vi "PrefDialog.vi"(8 "error in (no error)":errorcluster, 11 "MyPluginsBase in":refnum<class "PacificPowerSource.lvclass">) -> (0 "error out":errorcluster, 1 "Save As":bool, 2 "Changed":bool, 3 "MyPluginsBase out":refnum<class "PacificPowerSource.lvclass">)   [LabVIEW 2018, in "AcPwrPlugins.lvlib" / "PacificPowerSource.lvclass"]
doc: "This VI allows the user to load the previous device settings that were stored on disk via a .ini file, overwrite the device settings, and save the current settings to a completely new file."
uses:
  PacificPowerSource.lvclass
  C:/Users/Public/Documents/Projects/NistPluggableModules/AcPwr/AcPwrPlugins/AcPwrBaseClass/AcPwrBase.lvclass
  C:/Program Files (x86)/National Instruments/LabVIEW 2018/user.lib/NIST/BaseClasses/BasePlugin_class/BasePlugin.lvclass
  TypeDefs/LoadSettings.ctl
  TypeDefs/Measurements.ctl
  AcPwrBaseClass/AcPwrBase.lvclass/AcPwrBase.ctl
  FGen/MemberClasses/FunctionBaseClass/FunctionBase.lvclass
  <userlib>/NIST/BaseClasses/BasePlugin_class/BasePlugin.lvclass/BasePlugin.ctl
  AcPwrBaseClass/Accessors/Read RefreshTime.vi
  AcPwrBaseClass/Accessors/Read FunctionClass.vi
  AcPwrBaseClass/Accessors/Write FunctionClass.vi
  AcPwrBaseClass/Accessors/Write FunctionINIFilePath.vi
  <userlib>/NIST/BaseClasses/BasePlugin_class/Accessors/Read PluginIniFilePath.vi
  AcPwrBaseClass/Accessors/Write RefreshTime.vi
  <userlib>/NIST/BaseClasses/BasePlugin_class/Accessors/Write PluginIniFilePath.vi
  <vilib>/Utility/error.llb/Error Cluster From Error Code.vi
  <vilib>/ErrorRing/Error Ring.xnode
  <userlib>/NIST/BaseClasses/Object_class/BaseObject.lvclass
  <vilib>/Utility/config.llb/NI_LVConfig.lvlib
  AcPwrBaseClass/AcPwrBase.lvclass
panel:
  in  "Measurements":T1 {"Measurement Type (0: Voltage RMS L-N)" items=["Voltage RMS L-N", "Voltage RMS L-L", "Frequency", "Current RMS", "Current Peak", "Crest Factor", "Power Factor", "Power VA", "Real Power", "Voltage Harmonic THD", "Voltage Harmonic OHD", "Voltage Harmonic EHD", "Current Harmonic THD", "Current Harmonic OHD", "Current Harmonic EHD"]; "Channel Name(1: A)" items=["A"=1, "B"=2, "C"=3]}
  in  "WaveformIniFilePath":path
  in  "BtnConfigureWaveforms":bool
  in  "btnSaveAs":bool
  in  "RefreshTime":dbl
  in  "btnSave":bool
  in  "btnCancel":bool
  in  "Load Settings":T2 {"Arbitrary Waveform"."Waveform Number (2: Arbitrary Waveform2)" items=["Arbitrary Waveform 2"=2, "Arbitrary Waveform 3"=3, "Arbitrary Waveform 4"=4, "Arbitrary Waveform 5"=5, "Arbitrary Waveform 6"=6, "Arbitrary Waveform 7"=7, "Arbitrary Waveform 8"=8, "Arbitrary Waveform 9"=9, "Arbitrary Waveform 10"=10, "Arbitrary Waveform 11"=11, "Arbitrary Waveform 12"=12, "Arbitrary Waveform 13"=13, "Arbitrary Waveform 14"=14, "Arbitrary Waveform 15"=15, "Arbitrary Waveform 16"=16, "Arbitrary Waveform 17"=17, "Arbitrary Waveform 18"=18, "Arbitrary Waveform 19"=19, "Arbitrary Waveform 20"=20, "Arbitrary Waveform 21"=21, "Arbitrary Waveform 22"=22]; "Waveform"."Waveform (1: Sine)" items=["Sine"=1, "Arbitrary Waveform 2"=2, "Arbitrary Waveform 3"=3, "Arbitrary Waveform 4"=4, "Arbitrary Waveform 5"=5, "Arbitrary Waveform 6"=6, "Arbitrary Waveform 7"=7, "Arbitrary Waveform 8"=8, "Arbitrary Waveform 9"=9, "Arbitrary Waveform 10"=10, "Arbitrary Waveform 11"=11, "Arbitrary Waveform 12"=12, "Arbitrary Waveform 13"=13, "Arbitrary Waveform 14"=14, "Arbitrary Waveform 15"=15, "Arbitrary Waveform 16"=16, "Arbitrary Waveform 17"=17, "Arbitrary Waveform 18"=18, "Arbitrary Waveform 19"=19, "Arbitrary Waveform 20"=20, "Arbitrary Waveform 21"=21, "Arbitrary Waveform 22"=22]; "Waveform"."Channel Name (1: A)" items=["A"=1, "B"=2, "C"=3]; "Frequency"."Frequency Range (600Hz)" items=["150 Hz", "300 Hz", "600 Hz", "1200 Hz"]; "Range Control (0: Auto)" items=["Auto", "<110 V", "110 V -120.9 V", "121 V - 130.9 V", "> 131 V"]; "Configure Output"."Form (3: Three)" items=["Single", "Split", "Three"]; "Configure Output"."Coupling  (0: Direct)" items=["Direct", "Transformer"]}
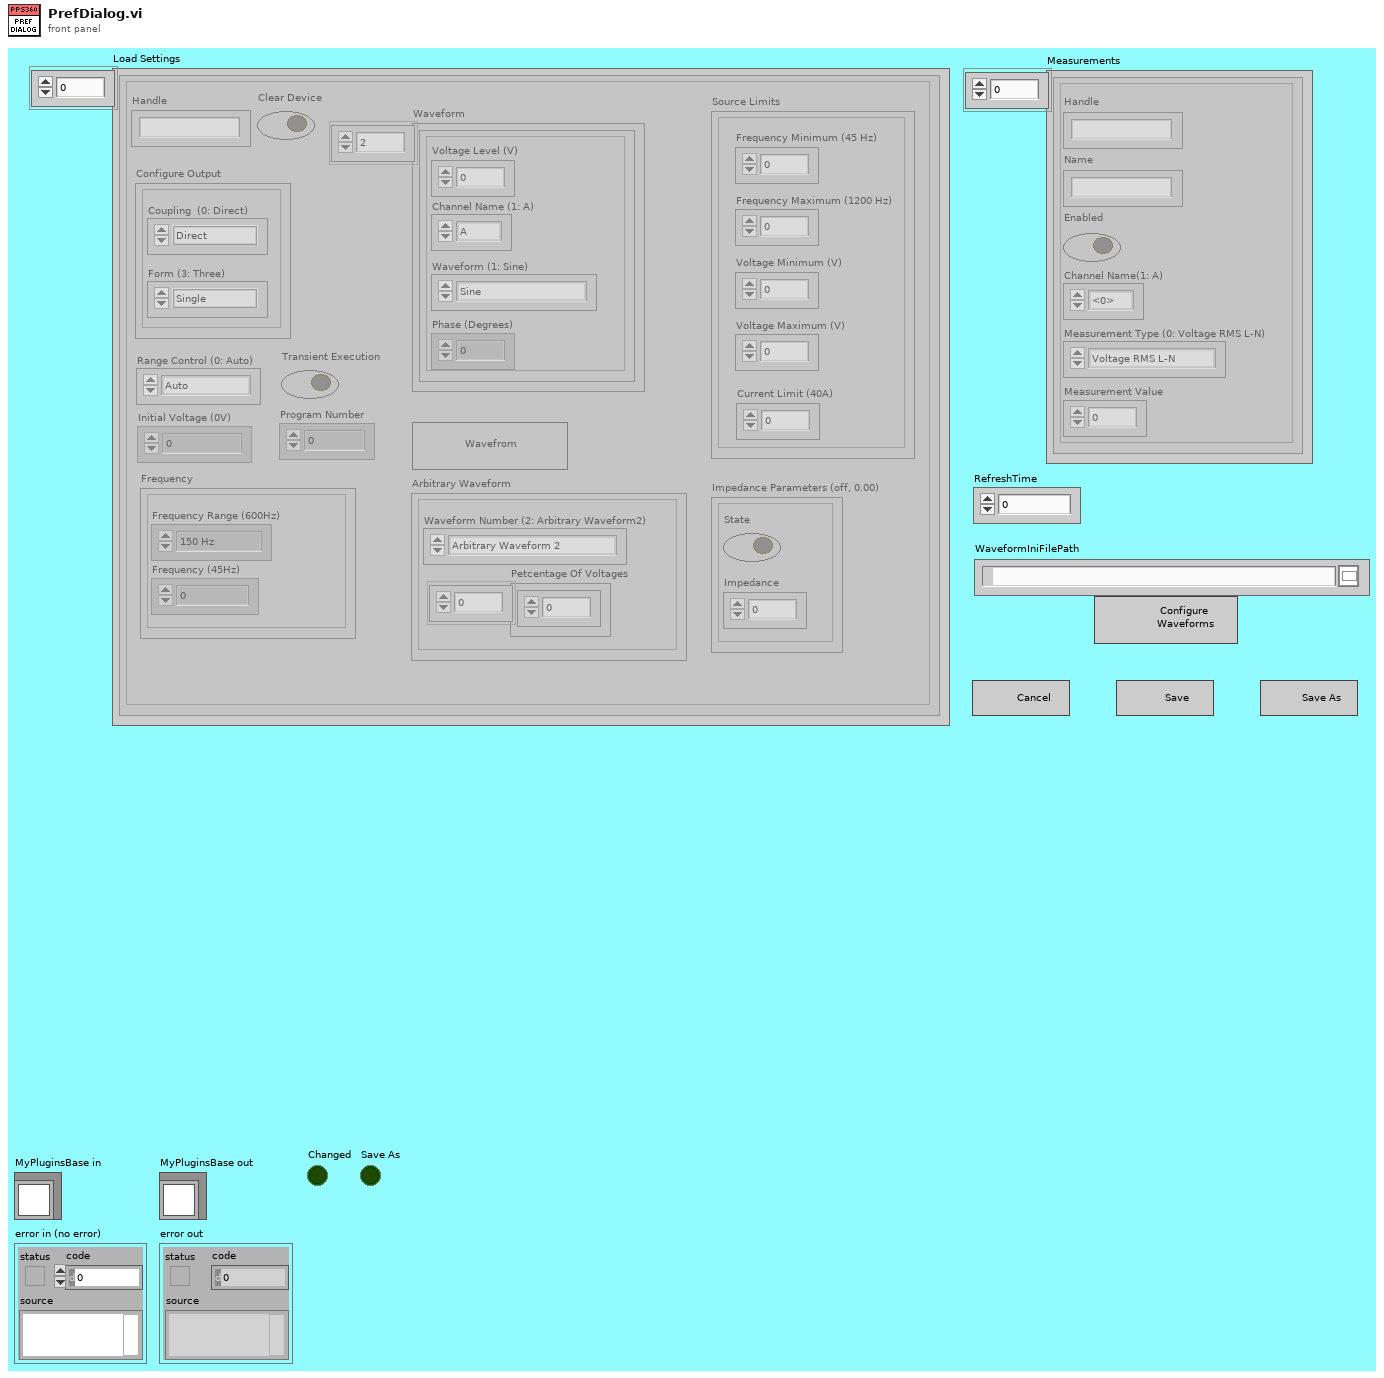
[diagram p1: front panel]
types:
  T1 = typedef "AcPwrPlugins.lvlib/PacificPowerSource.lvclass/Measurements.ctl" = cluster{"Handle":string, "Name":string, "Enabled":bool, "Measurement Value":dbl, "Channel Name(1: A)":u16, "Measurement Type (0: Voltage RMS L-N)":u16}[]
  T2 = typedef "AcPwrPlugins.lvlib/PacificPowerSource.lvclass/LoadSettings.ctl" = cluster{"Handle":string, "Connected":bool, "Source Limits":cluster{"Frequency Minimum (45 Hz)":dbl, "Frequency Maximum (1200 Hz)":dbl, "Voltage Maximum (V)":dbl, "Voltage Minimum (V)":dbl, "Current Limit (40A)":dbl}, "Clear Device":bool, "Configure Output":cluster{"Coupling  (0: Direct)":u16, "Form (3: Three)":u16}, "Range Control (0: Auto)":u16, "Initial Voltage (0V)":u16, "Frequency":cluster{"Frequency Range (600Hz)":u16, "Frequency (45Hz)":dbl}, "Waveform":cluster{"Voltage Level (V)":dbl, "Phase (Degrees)":i32, "Channel Name (1: A)":u16, "Waveform (1: Sine)":u16}[], "Arbitrary Waveform":cluster{"Waveform Number (2: Arbitrary Waveform2)":u16, "Petcentage Of Voltages":dbl[]}, "Impedance Parameters (off, 0.00)":cluster{"State":bool, "Impedance":dbl}, "Waveform Type":bool, "Program Number":i32, "Transient Execution":bool}[]
  T3 = enum32{"Invalid", "Standard", "Closed", "Hidden", "Minimized", "Maximized"}
  T4 = enum32{"Invalid", "Default", "Floating", "Floating/Auto-Hide", "Modal"}
  T5 = enum8{"Enabled", "Disabled", "Disabled and Grayed Out"}
  T6 = cluster{"Voltage Level (V)":dbl, "Phase (Degrees)":i32, "Channel Name (1: A)":u16, "Waveform (1: Sine)":u16}[]
  T7 = typedef "NI_LVConfig.lvlib/Config Data RefNum.ctl" = refnum<k1>
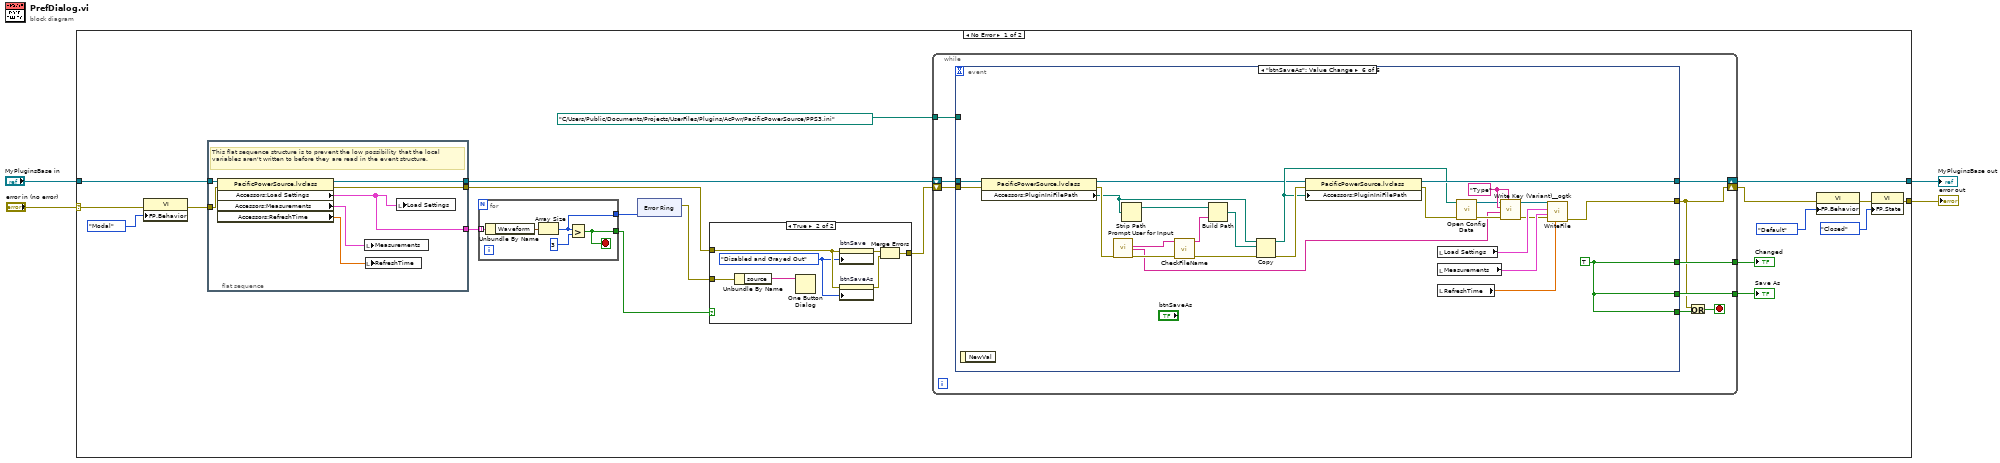
[diagram p0: block diagram]
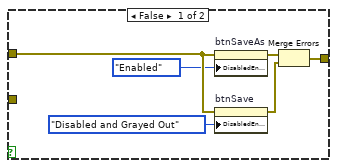
[diagram p2: hidden frame]
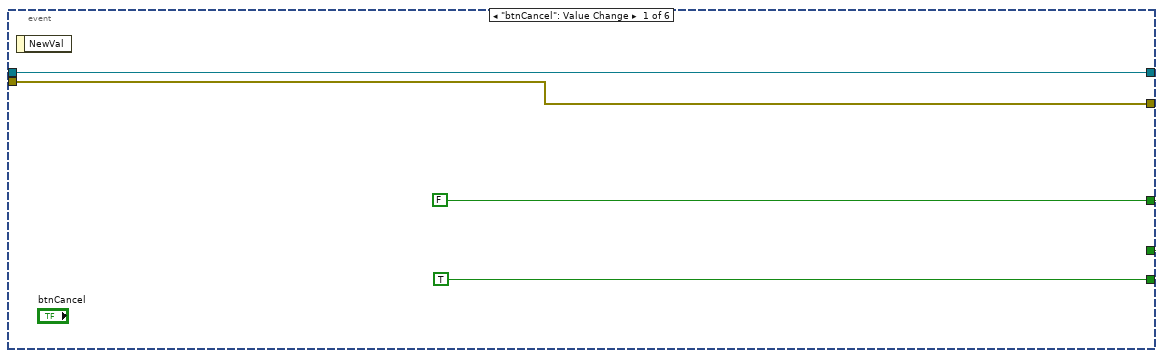
[diagram p3: hidden frame]
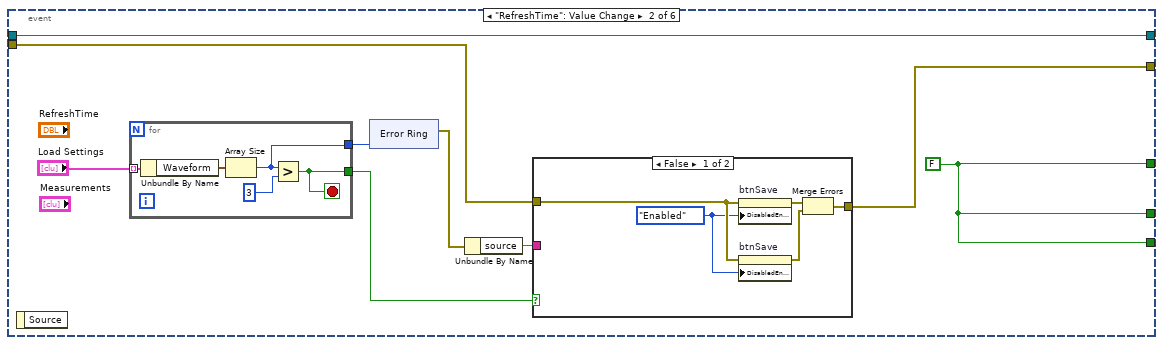
[diagram p4: hidden frame]
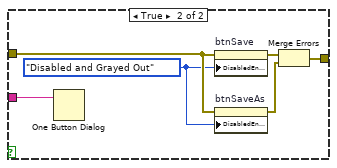
[diagram p5: hidden frame]
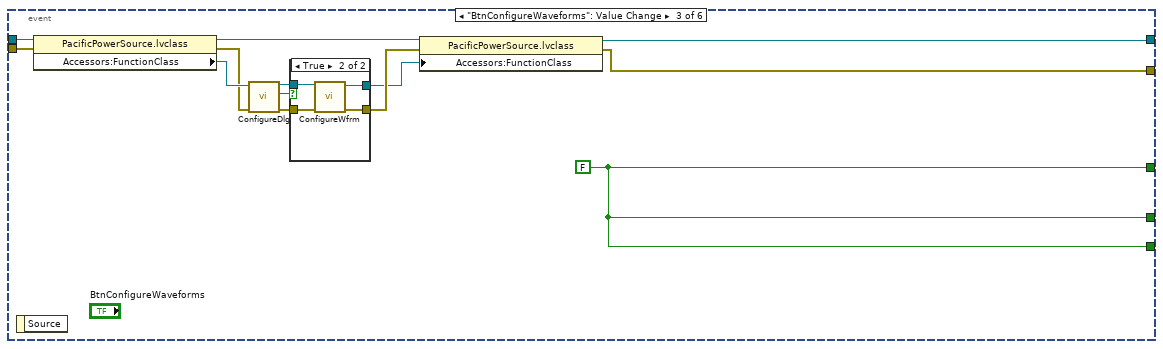
[diagram p6: hidden frame]
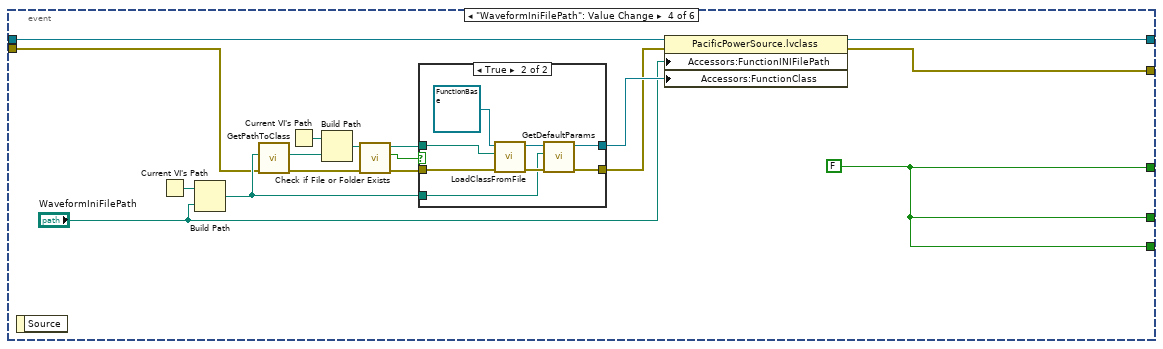
[diagram p8: hidden frame]
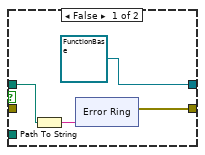
[diagram p9: hidden frame]
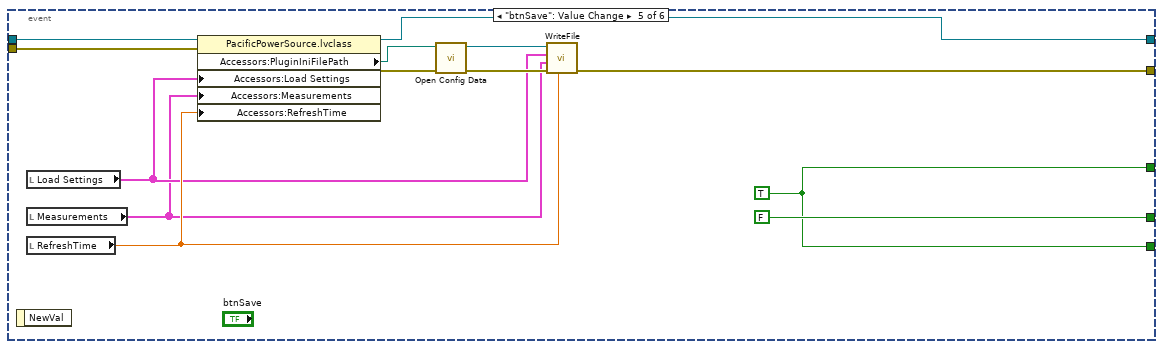
[diagram p10: hidden frame]
diagram:
  n1 = case shown="No Error" "error in (no error)" {
    selector: "error in (no error)" -> [w23 w197]
    tunnel: "MyPluginsBase in" -> [w18 w196]
    tunnel: [w16 w196] -> w2
    tunnel: [w15 w197] -> w1
    frame No Error {
      n2 = property class="VI"(error in=w23, "FP.Behavior"=T4."Modal" ("Front Panel Window:Behavior")) -> (error out=w19:errorcluster)  [unwired: 1 in, 1 out]
      n3 = flat-sequence {
        tunnel: w18 -> [w43]
        tunnel: [w42] -> w17
        tunnel: [w40] -> w7
        tunnel: w19 -> [w41]
        tunnel: [w37] -> w8
        frame #0 {
          # "This flat sequence structure is to prevent the low possibility that the local variables aren't written to before they are read in the event structure."
          n4 = property class="PacificPowerSource.lvclass"(reference=w43, error in=w41) -> (reference out=w42:refnum<class "PacificPowerSource.lvclass">, error out=w40:errorcluster, "Accessors:Load Settings"=w37:T2, "Accessors:Measurements"=w38:T1, "Accessors:RefreshTime"=w39:dbl)
          n5 = local write "Measurements"(w38) -> ()
          n6 = local write "RefreshTime"(w39) -> ()
          n7 = local write "Load Settings"(w37) -> ()
        }
      }
      n8 = for {
        tunnel: w8 -> [w34] mode=indexing
        tunnel: [w33] -> w10
        tunnel: [w32] -> w9
        stop <- w33 stop-if-true
        n9 = Unbundle By Name(w34) -> ("Waveform"=w36:T6)
        n10 = Array Size(array=w36) -> (size(s)=w32:i32)
        n11 = Greater?(x=w32, y=3) -> (0:w33:bool)
      }
      n12 = xnode "Error Ring"("parameter 0"=w9) -> ("error out"=w5:errorcluster)
      n13 = case shown="True" w10 {
        tunnel: w7 -> [w48 w55]
        tunnel: [w47 w54] -> w6
        tunnel: w5 -> [_ w51]
        frame False {
          # "Check if the number of Phases=Loads. If no disables the ability\nto save as."
          n14 = property on="btnSaveAs" class="Bool"(error in=w48, "DisabledEnum"=T5."Enabled" ("Disabled")) -> (error out=w49:errorcluster)  [unwired: 1 in, 1 out]
          n15 = property on="btnSave" class="Bool"(error in=w48, "DisabledEnum"=T5."Disabled and Grayed Out" ("Disabled")) -> (error out=w46:errorcluster)  [unwired: 1 in, 1 out]
          n16 = Merge Errors(w49, w46) -> (w47:errorcluster)
        }
        frame True {
          w52 = T5."Disabled and Grayed Out" ("Disabled")
          # "Check if the number of Phases=Loads. If no disables the ability\nto save as."
          n17 = Unbundle By Name(w51) -> ("source"=w50:string)
          n18 = One Button Dialog(message=w50) -> ()  [unwired: 1 in, 1 out]
          n19 = property on="btnSave" class="Bool"(error in=w55, "DisabledEnum"=w52) -> (error out=w56:errorcluster)  [unwired: 1 in, 1 out]
          n20 = property on="btnSaveAs" class="Bool"(error in=w55, "DisabledEnum"=w52) -> (error out=w53:errorcluster)  [unwired: 1 in, 1 out]
          n21 = Merge Errors(w56, w53) -> (w54:errorcluster)
        }
      }
      n22 = while {
        shift-right: [w62] -> w16
        shift-left: w17 -> [w63]
        tunnel: [w65] -> w12
        tunnel: [w60] -> w11
        tunnel: path "C:/Users/Public/Documents/Projects/UserFiles/Plugins/AcPwr/PacificPowerSource/PPS3.ini" ("Accessors:PluginIniFilePath") -> [w59]
        shift-right: [w57] -> w13
        shift-left: w6 -> [w61]
        stop <- w58 stop-if-true
        n23 = event shown="[5] \"btnSaveAs\": Value Change" {
          selector: _ -> [_ _ _ _ _ _]
          dyn-events: _ -> [_ _ _ _ _ _]
          timeout: _ -> [_ _ _ _ _ _]
          tunnel: [w66 w77 w102 w124 w165 w191] -> w65
          tunnel: [TRUE w77 w102 w124 w165 w191] -> w64
          tunnel: w63 -> [w68 w78 w106 w126 w168 w174]
          tunnel: [w68 w78 w103 w123 w164 w195] -> w62
          tunnel: [w67 w70 w104 w122 w161 w186] -> w57
          tunnel: w61 -> [w67 w71 w105 w125 w167 w173]
          tunnel: [w66 w77 w102 w124 FALSE w191] -> w60
          tunnel: w59 -> [_ _ _ _ _ _]
          event "btnCancel": Value Change {
            w66 = FALSE
            n24 = event-data() -> ()  [unwired: 1 in, 1 out]
          }
          event "RefreshTime": Value Change {
            w77 = FALSE
            n25 = event-data() -> ()  [unwired: 1 in, 1 out]
            n26 = for {
              tunnel: "Load Settings" -> [w88] mode=indexing
              tunnel: [w87] -> w76
              tunnel: [w86] -> w73
              stop <- w87 stop-if-true
              n27 = Unbundle By Name(w88) -> ("Waveform"=w90:T6)
              n28 = Array Size(array=w90) -> (size(s)=w86:i32)
              n29 = Greater?(x=w86, y=3) -> (0:w87:bool)
            }
            n30 = xnode "Error Ring"("parameter 0"=w73) -> ("error out"=w75:errorcluster)
            n31 = Unbundle By Name(w75) -> ("source"=w74:string)
            n32 = case shown="False" w76 {
              tunnel: w71 -> [w94 w100]
              tunnel: [w93 w99] -> w70
              tunnel: w74 -> [_ w96]
              frame False {
                w91 = T5."Enabled" ("Disabled")
                # "Check if the number of Phases=Loads. If no disables the ability\nto save as."
                n33 = property on="btnSave" class="Bool"(error in=w94, "DisabledEnum"=w91) -> (error out=w95:errorcluster)  [unwired: 1 in, 1 out]
                n34 = property on="btnSave" class="Bool"(error in=w94, "DisabledEnum"=w91) -> (error out=w92:errorcluster)  [unwired: 1 in, 1 out]
                n35 = Merge Errors(w95, w92) -> (w93:errorcluster)
              }
              frame True {
                w97 = T5."Disabled and Grayed Out" ("Disabled")
                # "Check if the number of Phases=Loads. If no disables the ability\nto save as."
                n36 = One Button Dialog(message=w96) -> ()  [unwired: 1 in, 1 out]
                n37 = property on="btnSave" class="Bool"(error in=w100, "DisabledEnum"=w97) -> (error out=w101:errorcluster)  [unwired: 1 in, 1 out]
                n38 = property on="btnSaveAs" class="Bool"(error in=w100, "DisabledEnum"=w97) -> (error out=w98:errorcluster)  [unwired: 1 in, 1 out]
                n39 = Merge Errors(w101, w98) -> (w99:errorcluster)
              }
            }
          }
          event "BtnConfigureWaveforms": Value Change {
            w102 = FALSE ("StartMeas")
            n40 = event-data() -> ()  [unwired: 1 in, 1 out]
            n41 = property class="PacificPowerSource.lvclass"(reference=w106, error in=w105) -> (reference out=w114:refnum<class "PacificPowerSource.lvclass">, error out=w108:errorcluster, "Accessors:FunctionClass"=w109:refnum<class "FunctionBase.lvclass">)
            n42 = call-dynamic "ConfigureDlg.vi"("error in (no error)"=w108, "FunctionBase in"=w109) -> ("error out"=w107:errorcluster, "Changed"=w111:bool, "FunctionBase out"=w110:refnum<class "FunctionBase.lvclass">)  [unwired: 7 in]
            n43 = case shown="True" w111 {
              tunnel: w107 -> [w115 w117]
              tunnel: w110 -> [w116 w120]
              tunnel: [w115 w119] -> w113
              tunnel: [w116 w118] -> w112
              frame False {
              }
              frame True {
                n44 = call-dynamic "ConfigureWfrm.vi"("error in (no error)"=w117, "FunctionBase in"=w120) -> ("error out"=w119:errorcluster, "FunctionBase out"=w118:refnum<class "FunctionBase.lvclass">)  [unwired: 8 in]
              }
            }
            n45 = property class="PacificPowerSource.lvclass"(reference=w114, error in=w113, "Accessors:FunctionClass"=w112) -> (reference out=w103:refnum<class "PacificPowerSource.lvclass">, error out=w104:errorcluster)
          }
          event "WaveformIniFilePath": Value Change {
            w124 = FALSE
            n46 = event-data() -> ()  [unwired: 1 in, 1 out]
            n47 = Current VI's Path() -> (path=w128:path)
            n48 = Build Path(base path=w128, name or relative path="WaveformIniFilePath") -> (appended path=w127:path)
            n49 = call <userlib>:"GetPathToClass.vi"("error in (no error)"=w125, "configuration file path"=w127) -> ("error IO"=w134:errorcluster, "PathToClass"=w136:path)  [unwired: 8 in]
            n50 = Current VI's Path() -> (path=w137:path)
            n51 = Build Path(base path=w137, name or relative path=w136) -> (appended path=w135:path)
            n52 = call <vilib>:"Check if File or Folder Exists.vi"("error in (no error)"=w134, "path"=w135) -> ("error out"=w131:errorcluster, "file or folder exists?"=w130:bool, "dup path"=w129:path)  [unwired: 7 in]
            n53 = case shown="True" w130 {
              tunnel: [w140 w151] -> w132
              tunnel: w131 -> [_ w156]
              tunnel: w129 -> [w139 w155]
              tunnel: [refnum<class "FunctionBase.lvclass"> refnum ("Functions.lvlib:FunctionBase.lvclass") w150] -> w133
              tunnel: w127 -> [_ w149]
              frame False {
                n54 = Path To String(path=w139) -> (string=w141:string)
                n55 = xnode "Error Ring"("parameter 0"=w141) -> ("error out"=w140:errorcluster)
              }
              frame True {
                n56 = call-dynamic "LoadClassFromFile.vi"("error in (no error)"=w156, "class path"=w155, "reference in"=refnum<class "FunctionBase.lvclass"> refnum ("Functions.lvlib:FunctionBase.lvclass")) -> ("error out"=w153:errorcluster, "reference out"=w152:refnum<class "FunctionBase.lvclass">)  [unwired: 7 in]
                n57 = call-dynamic "GetDefaultParams.vi"("error in (no error)"=w153, "Path"=w149, "FunctionBase in"=w152) -> ("error out"=w151:errorcluster, "FunctionBase out"=w150:refnum<class "FunctionBase.lvclass">)  [unwired: 7 in]
              }
            }
            n58 = property class="PacificPowerSource.lvclass"(reference=w126, error in=w132, "Accessors:FunctionINIFilePath"="WaveformIniFilePath", "Accessors:FunctionClass"=w133) -> (reference out=w123:refnum<class "PacificPowerSource.lvclass">, error out=w122:errorcluster)
          }
          event "btnSave": Value Change {
            w165 = TRUE ("StartMeas")
            n59 = event-data() -> ()  [unwired: 1 in, 1 out]
            n60 = local read "Load Settings"() -> (w159:T2)
            n61 = local read "Measurements"() -> (w158:T1)
            n62 = local read "RefreshTime"() -> (w162:dbl)
            n63 = property class="PacificPowerSource.lvclass"(reference=w168, error in=w167, "Accessors:Load Settings"=w159, "Accessors:Measurements"=w158, "Accessors:RefreshTime"=w162) -> (reference out=w164:refnum<class "PacificPowerSource.lvclass">, error out=w169:errorcluster, "Accessors:PluginIniFilePath"=w157:path)
            n64 = call <vilib>:"Open Config Data.vi"("error in (no error)"=w169, "configuration file path"=w157) -> ("error out"=w163:errorcluster, "refnum"=w160:T7)  [unwired: 7 in, 1 out]
            n65 = call "WriteFile.vi"("Refresh Time"=w162, "Error In"=w163, "Measurements"=w158, "Load Settings"=w159, "refnum"=w160) -> ("error out"=w161:errorcluster)  [unwired: 6 in]
          }
          event "btnSaveAs": Value Change {
            w180 = "Type" ("section (optional)")
            w191 = TRUE
            n66 = event-data() -> ()  [unwired: 1 in, 1 out]
            n67 = property class="PacificPowerSource.lvclass"(reference=w174, error in=w173) -> (reference out=w171:refnum<class "PacificPowerSource.lvclass">, error out=w172:errorcluster, "Accessors:PluginIniFilePath"=w170:path)
            n68 = call "Prompt User for Input"("error in (no error)"=w172) -> ("File Name"=w187:string, "PluginType"=w175:string, "error out"=w188:errorcluster)  [unwired: 15 in, 1 out]
            n69 = Strip Path(path=w170) -> (stripped path=w194:path)  [unwired: 1 out]
            n70 = call "CheckFileName.vi"("Error In"=w188, "File Name in"=w187) -> ("Error Out"=w189:errorcluster, "File Name out"=w190:string)  [unwired: 8 in]
            n71 = Build Path(base path=w194, name or relative path=w190) -> (appended path=w193:path)
            n72 = Copy(8:w189, 10:w193, 11:w170) -> (0:w192:errorcluster, 3:w181:path)  [unwired: 2 in, 1 out]
            n73 = property class="PacificPowerSource.lvclass"(reference=w171, error in=w192, "Accessors:PluginIniFilePath"=w181) -> (reference out=w195:refnum<class "PacificPowerSource.lvclass">, error out=w182:errorcluster)
            n74 = local read "Load Settings"() -> (w185:T2)
            n75 = local read "Measurements"() -> (w184:T1)
            n76 = local read "RefreshTime"() -> (w183:dbl)
            n77 = call <vilib>:"Open Config Data.vi"("error in (no error)"=w182, "configuration file path"=w181) -> ("error out"=w177:errorcluster, "refnum"=w178:T7)  [unwired: 7 in, 1 out]
            n78 = call <userlib>:"Write Key (Variant)__ogtk.vi"("section"=w180, "error in (no error)"=w177, "key-value"=w175, "key (optional)"=w180, "refnum"=w178) -> ("error out"=w176:errorcluster, "refnum out"=w179:T7)  [unwired: 5 in]
            n79 = call "WriteFile.vi"("Refresh Time"=w183, "Error In"=w176, "Measurements"=w184, "Load Settings"=w185, "refnum"=w179) -> ("error out"=w186:errorcluster)  [unwired: 6 in]
          }
        }
        n80 = Or(x=w57, y=w64) -> (x .or. y?=w58:bool)
      }
      "Save As" <- w11
      "Changed" <- w12
      n81 = property class="VI"(error in=w13, "FP.Behavior"=T4."Default" ("Front Panel Window:Behavior")) -> (error out=w22:errorcluster)  [unwired: 1 in, 1 out]
      n82 = property class="VI"(error in=w22, "FP.State"=T3."Closed" ("Front Panel Window:State")) -> (error out=w15:errorcluster)  [unwired: 1 in, 1 out]
    }
    frame Error {
    }
  }
  "error out" <- w1
  "MyPluginsBase out" <- w2
